vi "Failsafe.vi"(3 "Debug(NoSend)":bool, 4 "Body":string="Error", 5 "Password":string="labVIEW123", 6 "Email":string="krishna16842@gmail.com", 7 "Name of Experiment":string, 8 "error in":errorcluster, 9 "Emergency Contact (Carrier)":enum16{"T-Mobile", "AT&T", "Verizon", "Sprint"}(ring), 10 "Emergency Contact (phone number)":string, 11 "Process_REF":string) -> (0 "error out":errorcluster, 2 "Danger":bool)   [LabVIEW 2018]
uses:
  <vilib>/smtpClient/Set Message Text.vi
  <vilib>/smtpClient/LabVIEWSMTPClient.lvlib
panel:
  in  "TLS":bool=TRUE
  in  "Outgoing Mail Server (SMTP)":string="smtp.gmail.com"
  out "Path Out":path
  in  "Path In":path
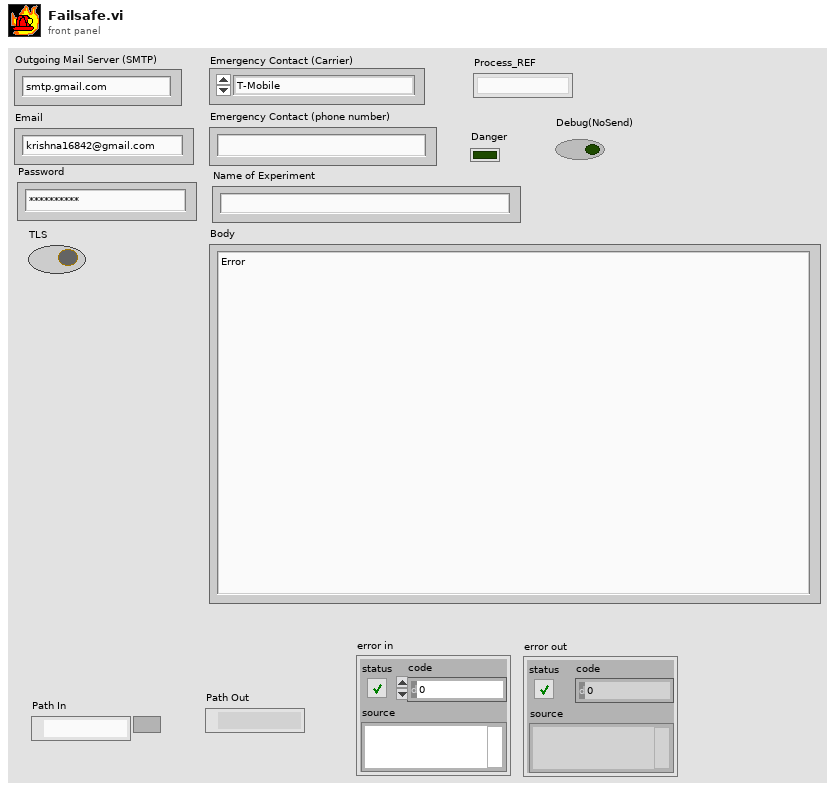
[diagram p1: front panel]
types:
  T1 = typedef "LabVIEWSMTPClient.lvlib/SmtpClientHandle.ctl" = refnum<k1>
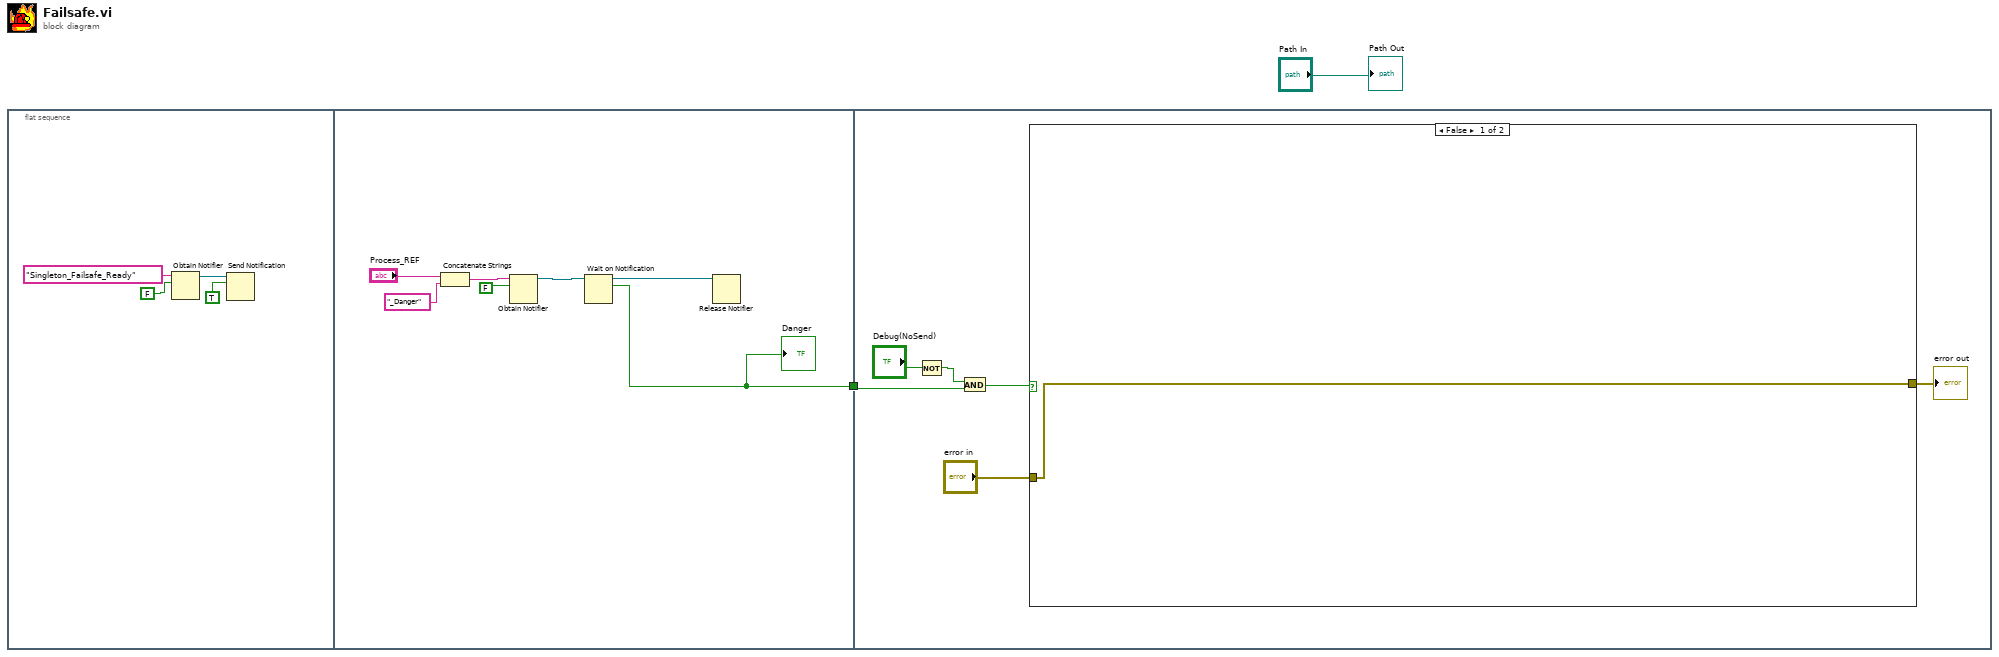
[diagram p0: block diagram]
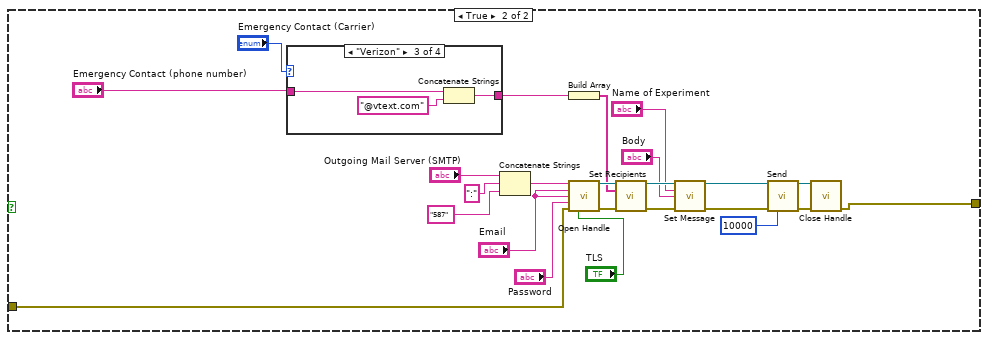
[diagram p2: hidden frame]
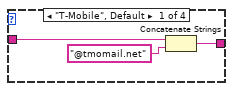
[diagram p3: hidden frame]
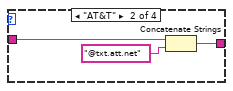
[diagram p4: hidden frame]
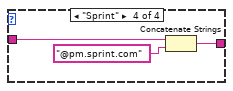
[diagram p5: hidden frame]
diagram:
  n1 = flat-sequence {
    tunnel: [w7] -> w1
    tunnel: w1 -> [w14]
    frame #0 {
      n2 = Obtain Notifier(name (unnamed)="Singleton_Failsafe_Ready", notification data type=FALSE) -> (notifier out=w3:refnum<notifier>)  [unwired: 2 in, 2 out]
      n3 = Send Notification(notification=TRUE, notifier=w3) -> ()  [unwired: 1 in, 2 out]
    }
    frame #1 {
      n4 = Concatenate Strings("Process_REF", "_Danger") -> (w11:string)
      n5 = Obtain Notifier(name (unnamed)=w11, notification data type=FALSE) -> (notifier out=w9:refnum<notifier>)  [unwired: 2 in, 2 out]
      n6 = Wait on Notification(notifier=w9) -> (notifier out=w8:refnum<notifier>, notification=w7:bool)  [unwired: 3 in, 2 out]
      "Danger" <- w7
      n7 = Release Notifier(notifier=w8) -> ()  [unwired: 2 in, 3 out]
    }
    frame #2 {
      n8 = Not(x="Debug(NoSend)") -> (.not. x?=w16:bool)
      n9 = And(x=w16, y=w14) -> (x .and. y?=w17:bool)
      n10 = case shown="False" w17 {
        tunnel: "error in" -> [w20 w22]
        tunnel: [w20 w21] -> w18
        frame False {
        }
        frame True {
          n11 = case shown="\"Verizon\"" "Emergency Contact (Carrier)" {
            tunnel: "Emergency Contact (phone number)" -> [w47 w49 w52 w55]
            tunnel: [w45 w50 w53 w56] -> w30
            frame "T-Mobile", Default {
              n12 = Concatenate Strings(w47, "@tmomail.net" ("string")) -> (w45:string)
            }
            frame "AT&T" {
              n13 = Concatenate Strings(w49, "@txt.att.net" ("string")) -> (w50:string)
            }
            frame "Verizon" {
              n14 = Concatenate Strings(w52, "@vtext.com" ("string")) -> (w53:string)
            }
            frame "Sprint" {
              n15 = Concatenate Strings(w55, "@pm.sprint.com") -> (w56:string)
            }
          }
          n16 = Concatenate Strings("Outgoing Mail Server (SMTP)", ":" ("string"), "587" ("Port")) -> (w25:string)
          n17 = Build Array(w30) -> (w29:string[])
          n18 = call <vilib>:"Open Handle.vi"("server address"=w25, "from"="Email", "username"="Email", "password"="Password", "error in (no error)"=w22, "use TLS (false)"="TLS") -> ("handle out"=w42:T1, "error out"=w39:errorcluster)  [unwired: 8 in]
          n19 = call <vilib>:"Set Recipients.vi"("handle in"=w42, "to"=w29, "error in (no error)"=w39) -> ("handle out"=w38:T1, "error out"=w37:errorcluster)  [unwired: 11 in]
          n20 = call-poly <vilib>:"Set Message.vi"("handle in"=w38, "subject"="Name of Experiment", "plain text message"="Body", "error in (no error)"=w37) -> ("handle out"=w34:T1, "error out"=w33:errorcluster)  [unwired: 10 in]
          n21 = call <vilib>:"Send.vi"("handle in"=w34, "error in (no error)"=w33, "timeout in ms (10000)"=10000) -> ("handle out"=w32:T1, "error out"=w31:errorcluster)  [unwired: 10 in, 1 out]
          n22 = call <vilib>:"Close Handle.vi"("handle in"=w32, "error in (no error)"=w31) -> ("error out"=w21:errorcluster)  [unwired: 12 in, 1 out]
        }
      }
      "error out" <- w18
    }
  }
  "Path Out" <- "Path In"
